vi "ge_XMLtoVarGrps.vi"(8 "error in":errorcluster, 10 "GXML String":string, 11 "ChanGroups":T1) -> (0 "error out":errorcluster, 2 "Speed Groups":T4[](array[typedef]))   [LabVIEW 2011]
uses:
  Custom Ctrls/Master Cfg/ge_ChanHeader.ctl
  Custom Ctrls/Master Cfg/ge_ChanDef.ctl
  Custom Ctrls/ge_MeasType.ctl
  Custom Ctrls/Master Cfg/ge_ChannelGroup.ctl
  Custom Ctrls/Master Cfg/ge_ChanVoltageCfg.ctl
  Custom Ctrls/Master CfgXML/ge_VoltChan.ctl
  Custom Ctrls/Master CfgXML/ge_VoltGroup.ctl
  Custom Ctrls/Master Cfg/ge_ChanDynamicCfg.ctl
  Custom Ctrls/Master CfgXML/ge_DyanChan.ctl
  Custom Ctrls/Master CfgXML/ge_DynGroup.ctl
  Custom Ctrls/Master Cfg/ge_ChanThrmcplCfg.ctl
  Custom Ctrls/Master CfgXML/ge_ThrmcplChan.ctl
  Custom Ctrls/Master CfgXML/ge_ThrmcplGroup.ctl
  Custom Ctrls/Master Cfg/ge_ChanRTDCfg.ctl
  Custom Ctrls/Master CfgXML/ge_RTDChan.ctl
  Custom Ctrls/Master CfgXML/ge_RTDGroup.ctl
  Custom Ctrls/Master Cfg/ge_ChanStrainCfg.ctl
  Custom Ctrls/Master CfgXML/ge_StrainChan.ctl
  Custom Ctrls/Master CfgXML/ge_StrainGroup.ctl
  Custom Ctrls/Master CfgXML/ge_CurrentChan.ctl
  Custom Ctrls/Master CfgXML/ge_CurrentGroup.ctl
  Custom Ctrls/Master Cfg/ge_ChanResCfg.ctl
  Custom Ctrls/Master CfgXML/ge_ResChan.ctl
  Custom Ctrls/Master CfgXML/ge_ResGroup.ctl
  Custom Ctrls/Master Cfg/ge_ChanFreqCfg.ctl
  Custom Ctrls/Master CfgXML/ge_FreqChan.ctl
  Custom Ctrls/Master CfgXML/ge_FreqGroup.ctl
  Custom Ctrls/Master Cfg/ge_ChanCurrentCfg.ctl
  Custom Ctrls/Master CfgXML/ge_TachGroup.ctl
  Custom Ctrls/Master CfgXML/ge_TachChan.ctl
  Custom Ctrls/Master Cfg/ge_ChanTachCfg.ctl
  Custom Ctrls/Master Cfg/ge_TachProcess.ctl
  Classes/Channel/Channel.lvclass
  Custom Ctrls/Master Cfg/ge_GrpHdr.ctl
  Custom Ctrls/Master CfgXML/ge_XMLHdr_ChanGroups.ctl
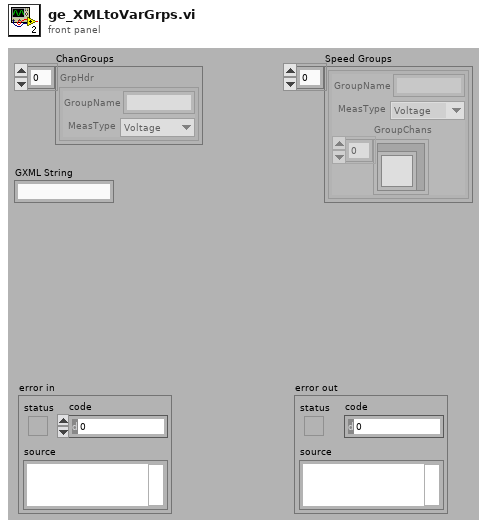
[diagram p1: front panel]
types:
  T1 = typedef "ge_XMLHdr_ChanGroups.ctl" = T2[]
  T2 = typedef "ge_GrpHdr.ctl" = cluster{"GroupName":string, "MeasType":T3}
  T3 = typedef "ge_MeasType.ctl" = enum16{"Voltage", "Frequency", "Tachometer", "Dynamic", "Thermocouple", "RTD", "Strain", "Current", "Resistance"}
  T4 = typedef "ge_ChannelGroup.ctl" = cluster{"GroupName":string, "MeasType":T3, "GroupChans":refnum<class "Channel.lvclass">[]}
  T5 = typedef "ge_VoltGroup.ctl" = cluster{"GroupName":string, "MeasType":T3, "GroupMems":T6[]}
  T6 = typedef "ge_VoltChan.ctl" = cluster{"ChanHdr":T7, "VoltChanCfg":T8}
  T7 = typedef "ge_ChanHeader.ctl" = cluster{"ChanName":string, "Alias":string, "ModbusAddr":string, "Device":string, "ToModBus":bool}
  T8 = typedef "ge_ChanVoltageCfg.ctl" = cluster{"VRange":dbl, "Term Cfg":u16, "Coupling":u16, "Scale":dbl, "Offset":dbl, "Unit_EU":string}
  T9 = typedef "ge_ChanDef.ctl" = cluster{"ChanHdr":T7, "ChanCfg":variant}
  T10 = typedef "ge_FreqGroup.ctl" = cluster{"GroupName":string, "MeasType":T3, "GroupMems":T11[]}
  T11 = typedef "ge_FreqChan.ctl" = cluster{"ChanHdr":T7, "FreqChanCfg":T12}
  T12 = typedef "ge_ChanFreqCfg.ctl" = cluster{"VRange":dbl, "Term Cfg":u16, "Coupling":u16, "Thresh":dbl, "Slope":u16, "Min EU":dbl, "Scale":dbl, "Offset":dbl, "Unit_EU":string}
  T13 = typedef "ge_TachGroup.ctl" = cluster{"GroupName":string, "MeasType":T3, "GroupMems":T14[]}
  T14 = typedef "ge_TachChan.ctl" = cluster{"ChanHdr":T7, "TachChanCfg":T15}
  T15 = typedef "ge_ChanTachCfg.ctl" = cluster{"VRange":dbl, "Term Cfg":u16, "Coupling":u16, "Unit_EU":string, "TachProc":T16}
  T16 = typedef "ge_TachProcess.ctl" = cluster{"PPR":dbl, "Thresh_V":dbl, "Slope":u16, "MinRPM":dbl}
  T17 = typedef "ge_DynGroup.ctl" = cluster{"GroupName":string, "MeasType":T3, "GroupMems":T18[]}
  T18 = typedef "ge_DyanChan.ctl" = cluster{"ChanHdr":T7, "DynChanCfg":T19}
  T19 = typedef "ge_ChanDynamicCfg.ctl" = cluster{"Sensitivity":dbl, "Unit_EU":string, "Iex":dbl, "VRange":dbl, "dB":bool, "dB Ref":dbl, "Cal Mag":dbl, "Cal Units":u16}
  T20 = typedef "ge_ThrmcplGroup.ctl" = cluster{"GroupName":string, "MeasType":T3, "GroupMems":T21[]}
  T21 = typedef "ge_ThrmcplChan.ctl" = cluster{"ChanHdr":T7, "ThrmcplChanCfg":T22}
  T22 = typedef "ge_ChanThrmcplCfg.ctl" = cluster{"Units":u16, "Type":u16, "cjc source":u16, "cjc val":dbl, "Scale":dbl, "Offset":dbl, "Approx Max":i32, "Approx Min":i32}
  T23 = typedef "ge_RTDGroup.ctl" = cluster{"GroupName":string, "MeasType":T3, "GroupMems":T24[]}
  T24 = typedef "ge_RTDChan.ctl" = cluster{"ChanHdr":T7, "RTDChanCfg":T25}
  T25 = typedef "ge_ChanRTDCfg.ctl" = cluster{"Ro":u16, "Units":u16, "Type":u16, "WireCfg":u16, "Scale":dbl, "Offset":dbl, "Approx Max":i32, "Approx Min":i32}
  T26 = typedef "ge_StrainGroup.ctl" = cluster{"GroupName":string, "MeasType":T3, "GroupMems":T27[]}
  T27 = typedef "ge_StrainChan.ctl" = cluster{"ChanHdr":T7, "StrainChanCfg":T28}
  T28 = typedef "ge_ChanStrainCfg.ctl" = cluster{"Strain Mode":u16, "Vex":dbl, "Bridge Type":u16, "GF":dbl, "Gauge Res":i32, "Poisson":dbl, "Lead Res":dbl, "Init uStrain":dbl, "GAF":dbl, "Approx Max":dbl, "Approx Min":dbl}
  T29 = typedef "ge_CurrentGroup.ctl" = cluster{"GroupName":string, "MeasType":T3, "GroupMems":T30[]}
  T30 = typedef "ge_CurrentChan.ctl" = cluster{"ChanHdr":T7, "CurrentChanCfg":T31}
  T31 = typedef "ge_ChanCurrentCfg.ctl" = cluster{"IRange":dbl, "Scale":dbl, "Offset":dbl, "Unit_EU":string}
  T32 = typedef "ge_ResGroup.ctl" = cluster{"GroupName":string, "MeasType":T3, "GroupMems":T33[]}
  T33 = typedef "ge_ResChan.ctl" = cluster{"ChanHdr":T7, "ResChanCfg":T34}
  T34 = typedef "ge_ChanResCfg.ctl" = cluster{"ORange":u16, "WireCfg":u16, "Scale":dbl, "Offset":dbl, "Unit_EU":string}
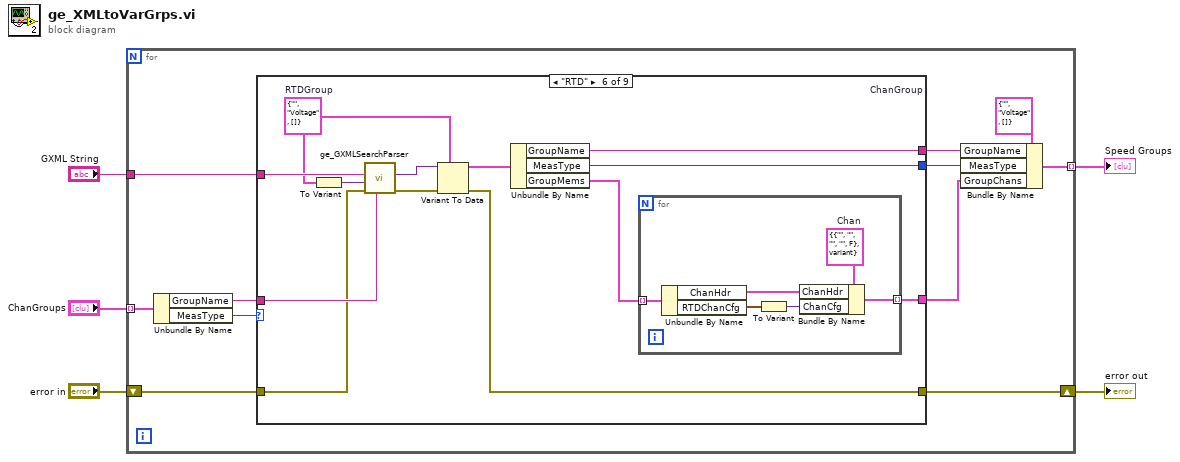
[diagram p0: block diagram]
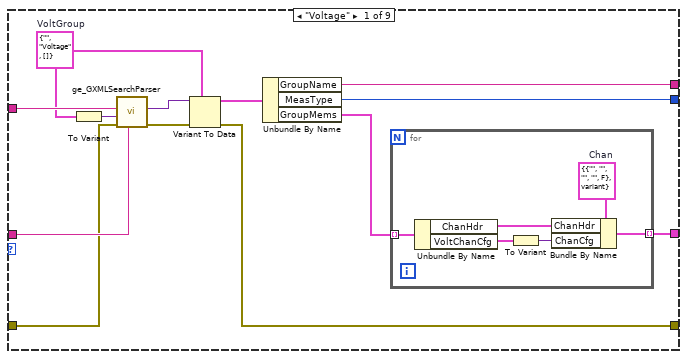
[diagram p2: hidden frame]
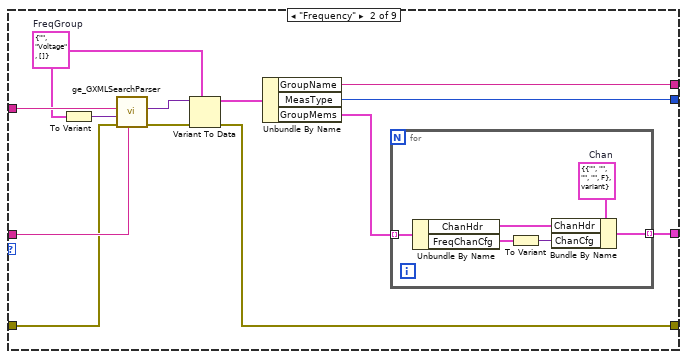
[diagram p3: hidden frame]
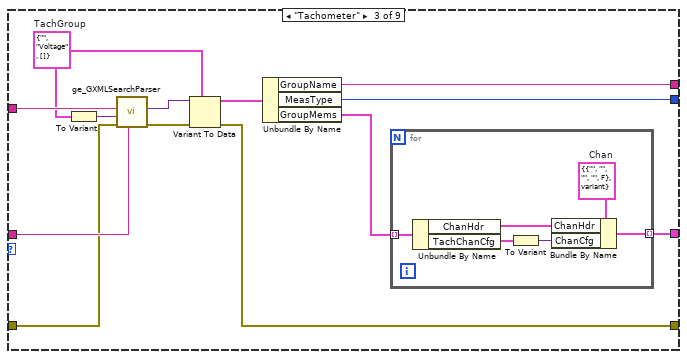
[diagram p4: hidden frame]
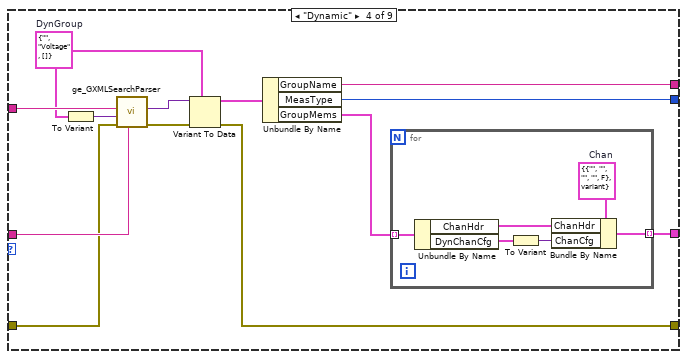
[diagram p5: hidden frame]
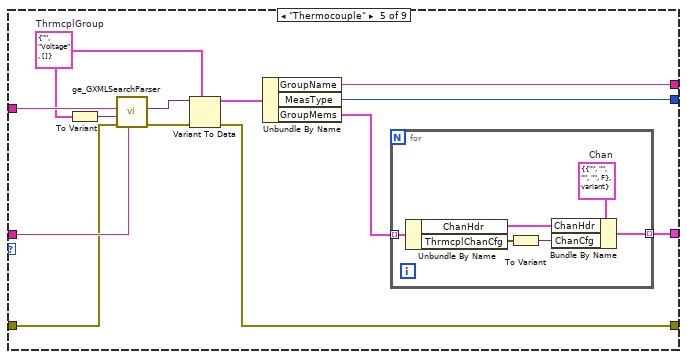
[diagram p6: hidden frame]
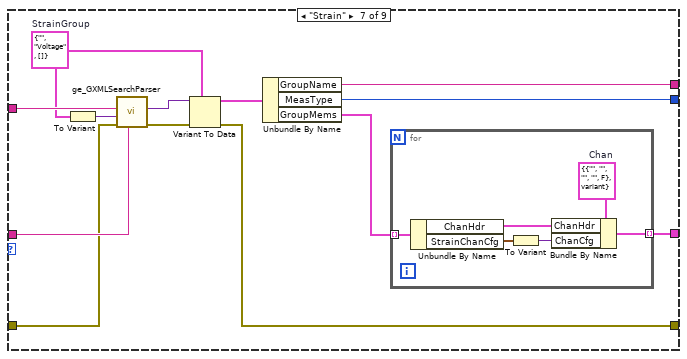
[diagram p7: hidden frame]
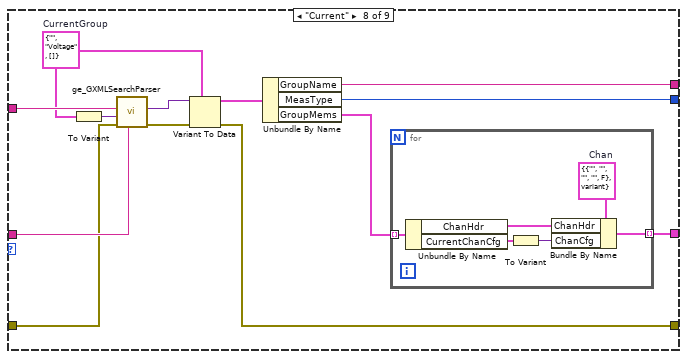
[diagram p8: hidden frame]
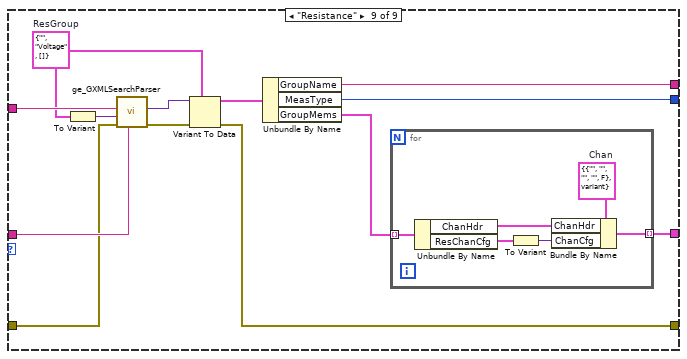
[diagram p9: hidden frame]
diagram:
  n1 = for {
    tunnel: "ChanGroups" -> [w16] mode=indexing
    tunnel: "GXML String" -> [w14]
    shift-right: [w12] -> w5
    shift-left: "error in" -> [w13]
    tunnel: [w6] -> w4 mode=indexing
    w10 = T4 {"GroupName"="", "MeasType"=enum."Voltage", "GroupChans"=[]}  # ChanGroup
    n2 = Unbundle By Name(w16) -> ("GroupName"=w15:string, "MeasType"=w11:T3)
    n3 = case shown="\"RTD\"" w11 {
      tunnel: w15 -> [w29 w48 w67 w86 w105 w124 w143 w162 w181]
      tunnel: w14 -> [w28 w47 w66 w85 w104 w123 w142 w161 w180]
      tunnel: w13 -> [w27 w46 w65 w84 w103 w122 w141 w160 w179]
      tunnel: [w24 w43 w62 w81 w100 w119 w138 w157 w176] -> w12
      tunnel: [w21 w40 w59 w78 w97 w116 w135 w154 w173] -> w9
      tunnel: [w20 w39 w58 w77 w96 w115 w134 w153 w172] -> w8
      tunnel: [w19 w38 w57 w76 w95 w114 w133 w152 w171] -> w7
      frame "Voltage" {
        w17 = T5 {"GroupName"="", "MeasType"=enum."Voltage", "GroupMems"=[]}  # VoltGroup
        n4 = To Variant(anything=w17) -> (Variant=w18:variant)
        n5 = call "ge_GXMLSearchParser.vi"("String ID"=w29, "error in"=w27, "TypeDesc"=w18, "XML String In"=w28) -> ("error out"=w25:errorcluster, "Parsed Data"=w26:variant)  [unwired: 6 in]
        n6 = Variant To Data(error in=w25, type=w17, Variant=w26) -> (data=w23:T5, error out=w24:errorcluster)
        n7 = Unbundle By Name(w23) -> ("GroupName"=w21:string, "MeasType"=w20:T3, "GroupMems"=w22:T6[])
        n8 = for {
          tunnel: w22 -> [w35] mode=indexing
          tunnel: [w30] -> w19 mode=indexing
          w33 = T9 {"ChanHdr"={"ChanName"="", "Alias"="", "ModbusAddr"="", "Device"="", "ToModBus"=FALSE}, "ChanCfg"=variant}  # Chan
          n9 = Unbundle By Name(w35) -> ("ChanHdr"=w32:T7, "VoltChanCfg"=w34:T8)
          n10 = To Variant(anything=w34) -> (Variant=w31:variant)
          n11 = Bundle By Name(cluster=w33, "ChanHdr"=w32, "ChanCfg"=w31) -> (w30:T9)
        }
      }
      frame "Frequency" {
        w36 = T10 {"GroupName"="", "MeasType"=enum."Voltage", "GroupMems"=[]}  # FreqGroup
        n12 = To Variant(anything=w36) -> (Variant=w37:variant)
        n13 = call "ge_GXMLSearchParser.vi"("String ID"=w48, "error in"=w46, "TypeDesc"=w37, "XML String In"=w47) -> ("error out"=w44:errorcluster, "Parsed Data"=w45:variant)  [unwired: 6 in]
        n14 = Variant To Data(error in=w44, type=w36, Variant=w45) -> (data=w42:T10, error out=w43:errorcluster)
        n15 = Unbundle By Name(w42) -> ("GroupName"=w40:string, "MeasType"=w39:T3, "GroupMems"=w41:T11[])
        n16 = for {
          tunnel: w41 -> [w54] mode=indexing
          tunnel: [w49] -> w38 mode=indexing
          w52 = T9 {"ChanHdr"={"ChanName"="", "Alias"="", "ModbusAddr"="", "Device"="", "ToModBus"=FALSE}, "ChanCfg"=variant}  # Chan
          n17 = Unbundle By Name(w54) -> ("ChanHdr"=w51:T7, "FreqChanCfg"=w53:T12)
          n18 = To Variant(anything=w53) -> (Variant=w50:variant)
          n19 = Bundle By Name(cluster=w52, "ChanHdr"=w51, "ChanCfg"=w50) -> (w49:T9)
        }
      }
      frame "Tachometer" {
        w55 = T13 {"GroupName"="", "MeasType"=enum."Voltage", "GroupMems"=[]}  # TachGroup
        n20 = To Variant(anything=w55) -> (Variant=w56:variant)
        n21 = call "ge_GXMLSearchParser.vi"("String ID"=w67, "error in"=w65, "TypeDesc"=w56, "XML String In"=w66) -> ("error out"=w63:errorcluster, "Parsed Data"=w64:variant)  [unwired: 6 in]
        n22 = Variant To Data(error in=w63, type=w55, Variant=w64) -> (data=w61:T13, error out=w62:errorcluster)
        n23 = Unbundle By Name(w61) -> ("GroupName"=w59:string, "MeasType"=w58:T3, "GroupMems"=w60:T14[])
        n24 = for {
          tunnel: w60 -> [w73] mode=indexing
          tunnel: [w68] -> w57 mode=indexing
          w71 = T9 {"ChanHdr"={"ChanName"="", "Alias"="", "ModbusAddr"="", "Device"="", "ToModBus"=FALSE}, "ChanCfg"=variant}  # Chan
          n25 = Unbundle By Name(w73) -> ("ChanHdr"=w70:T7, "TachChanCfg"=w72:T15)
          n26 = To Variant(anything=w72) -> (Variant=w69:variant)
          n27 = Bundle By Name(cluster=w71, "ChanHdr"=w70, "ChanCfg"=w69) -> (w68:T9)
        }
      }
      frame "Dynamic" {
        w74 = T17 {"GroupName"="", "MeasType"=enum."Voltage", "GroupMems"=[]}  # DynGroup
        n28 = To Variant(anything=w74) -> (Variant=w75:variant)
        n29 = call "ge_GXMLSearchParser.vi"("String ID"=w86, "error in"=w84, "TypeDesc"=w75, "XML String In"=w85) -> ("error out"=w82:errorcluster, "Parsed Data"=w83:variant)  [unwired: 6 in]
        n30 = Variant To Data(error in=w82, type=w74, Variant=w83) -> (data=w80:T17, error out=w81:errorcluster)
        n31 = Unbundle By Name(w80) -> ("GroupName"=w78:string, "MeasType"=w77:T3, "GroupMems"=w79:T18[])
        n32 = for {
          tunnel: w79 -> [w92] mode=indexing
          tunnel: [w87] -> w76 mode=indexing
          w90 = T9 {"ChanHdr"={"ChanName"="", "Alias"="", "ModbusAddr"="", "Device"="", "ToModBus"=FALSE}, "ChanCfg"=variant}  # Chan
          n33 = Unbundle By Name(w92) -> ("ChanHdr"=w89:T7, "DynChanCfg"=w91:T19)
          n34 = To Variant(anything=w91) -> (Variant=w88:variant)
          n35 = Bundle By Name(cluster=w90, "ChanHdr"=w89, "ChanCfg"=w88) -> (w87:T9)
        }
      }
      frame "Thermocouple" {
        w93 = T20 {"GroupName"="", "MeasType"=enum."Voltage", "GroupMems"=[]}  # ThrmcplGroup
        n36 = To Variant(anything=w93) -> (Variant=w94:variant)
        n37 = call "ge_GXMLSearchParser.vi"("String ID"=w105, "error in"=w103, "TypeDesc"=w94, "XML String In"=w104) -> ("error out"=w101:errorcluster, "Parsed Data"=w102:variant)  [unwired: 6 in]
        n38 = Variant To Data(error in=w101, type=w93, Variant=w102) -> (data=w99:T20, error out=w100:errorcluster)
        n39 = Unbundle By Name(w99) -> ("GroupName"=w97:string, "MeasType"=w96:T3, "GroupMems"=w98:T21[])
        n40 = for {
          tunnel: w98 -> [w111] mode=indexing
          tunnel: [w106] -> w95 mode=indexing
          w109 = T9 {"ChanHdr"={"ChanName"="", "Alias"="", "ModbusAddr"="", "Device"="", "ToModBus"=FALSE}, "ChanCfg"=variant}  # Chan
          n41 = Unbundle By Name(w111) -> ("ChanHdr"=w108:T7, "ThrmcplChanCfg"=w110:T22)
          n42 = To Variant(anything=w110) -> (Variant=w107:variant)
          n43 = Bundle By Name(cluster=w109, "ChanHdr"=w108, "ChanCfg"=w107) -> (w106:T9)
        }
      }
      frame "RTD" {
        w112 = T23 {"GroupName"="", "MeasType"=enum."Voltage", "GroupMems"=[]}  # RTDGroup
        n44 = To Variant(anything=w112) -> (Variant=w113:variant)
        n45 = call "ge_GXMLSearchParser.vi"("String ID"=w124, "error in"=w122, "TypeDesc"=w113, "XML String In"=w123) -> ("error out"=w120:errorcluster, "Parsed Data"=w121:variant)  [unwired: 6 in]
        n46 = Variant To Data(error in=w120, type=w112, Variant=w121) -> (data=w118:T23, error out=w119:errorcluster)
        n47 = Unbundle By Name(w118) -> ("GroupName"=w116:string, "MeasType"=w115:T3, "GroupMems"=w117:T24[])
        n48 = for {
          tunnel: w117 -> [w130] mode=indexing
          tunnel: [w125] -> w114 mode=indexing
          w128 = T9 {"ChanHdr"={"ChanName"="", "Alias"="", "ModbusAddr"="", "Device"="", "ToModBus"=FALSE}, "ChanCfg"=variant}  # Chan
          n49 = Unbundle By Name(w130) -> ("ChanHdr"=w127:T7, "RTDChanCfg"=w129:T25)
          n50 = To Variant(anything=w129) -> (Variant=w126:variant)
          n51 = Bundle By Name(cluster=w128, "ChanHdr"=w127, "ChanCfg"=w126) -> (w125:T9)
        }
      }
      frame "Strain" {
        w131 = T26 {"GroupName"="", "MeasType"=enum."Voltage", "GroupMems"=[]}  # StrainGroup
        n52 = To Variant(anything=w131) -> (Variant=w132:variant)
        n53 = call "ge_GXMLSearchParser.vi"("String ID"=w143, "error in"=w141, "TypeDesc"=w132, "XML String In"=w142) -> ("error out"=w139:errorcluster, "Parsed Data"=w140:variant)  [unwired: 6 in]
        n54 = Variant To Data(error in=w139, type=w131, Variant=w140) -> (data=w137:T26, error out=w138:errorcluster)
        n55 = Unbundle By Name(w137) -> ("GroupName"=w135:string, "MeasType"=w134:T3, "GroupMems"=w136:T27[])
        n56 = for {
          tunnel: w136 -> [w149] mode=indexing
          tunnel: [w144] -> w133 mode=indexing
          w147 = T9 {"ChanHdr"={"ChanName"="", "Alias"="", "ModbusAddr"="", "Device"="", "ToModBus"=FALSE}, "ChanCfg"=variant}  # Chan
          n57 = Unbundle By Name(w149) -> ("ChanHdr"=w146:T7, "StrainChanCfg"=w148:T28)
          n58 = To Variant(anything=w148) -> (Variant=w145:variant)
          n59 = Bundle By Name(cluster=w147, "ChanHdr"=w146, "ChanCfg"=w145) -> (w144:T9)
        }
      }
      frame "Current" {
        w150 = T29 {"GroupName"="", "MeasType"=enum."Voltage", "GroupMems"=[]}  # CurrentGroup
        n60 = To Variant(anything=w150) -> (Variant=w151:variant)
        n61 = call "ge_GXMLSearchParser.vi"("String ID"=w162, "error in"=w160, "TypeDesc"=w151, "XML String In"=w161) -> ("error out"=w158:errorcluster, "Parsed Data"=w159:variant)  [unwired: 6 in]
        n62 = Variant To Data(error in=w158, type=w150, Variant=w159) -> (data=w156:T29, error out=w157:errorcluster)
        n63 = Unbundle By Name(w156) -> ("GroupName"=w154:string, "MeasType"=w153:T3, "GroupMems"=w155:T30[])
        n64 = for {
          tunnel: w155 -> [w168] mode=indexing
          tunnel: [w163] -> w152 mode=indexing
          w166 = T9 {"ChanHdr"={"ChanName"="", "Alias"="", "ModbusAddr"="", "Device"="", "ToModBus"=FALSE}, "ChanCfg"=variant}  # Chan
          n65 = Unbundle By Name(w168) -> ("ChanHdr"=w165:T7, "CurrentChanCfg"=w167:T31)
          n66 = To Variant(anything=w167) -> (Variant=w164:variant)
          n67 = Bundle By Name(cluster=w166, "ChanHdr"=w165, "ChanCfg"=w164) -> (w163:T9)
        }
      }
      frame "Resistance" {
        w169 = T32 {"GroupName"="", "MeasType"=enum."Voltage", "GroupMems"=[]}  # ResGroup
        n68 = To Variant(anything=w169) -> (Variant=w170:variant)
        n69 = call "ge_GXMLSearchParser.vi"("String ID"=w181, "error in"=w179, "TypeDesc"=w170, "XML String In"=w180) -> ("error out"=w177:errorcluster, "Parsed Data"=w178:variant)  [unwired: 6 in]
        n70 = Variant To Data(error in=w177, type=w169, Variant=w178) -> (data=w175:T32, error out=w176:errorcluster)
        n71 = Unbundle By Name(w175) -> ("GroupName"=w173:string, "MeasType"=w172:T3, "GroupMems"=w174:T33[])
        n72 = for {
          tunnel: w174 -> [w187] mode=indexing
          tunnel: [w182] -> w171 mode=indexing
          w185 = T9 {"ChanHdr"={"ChanName"="", "Alias"="", "ModbusAddr"="", "Device"="", "ToModBus"=FALSE}, "ChanCfg"=variant}  # Chan
          n73 = Unbundle By Name(w187) -> ("ChanHdr"=w184:T7, "ResChanCfg"=w186:T34)
          n74 = To Variant(anything=w186) -> (Variant=w183:variant)
          n75 = Bundle By Name(cluster=w185, "ChanHdr"=w184, "ChanCfg"=w183) -> (w182:T9)
        }
      }
    }
    n76 = Bundle By Name(cluster=w10, "GroupName"=w9, "MeasType"=w8, "GroupChans"=w7) -> (w6:T4)
  }
  "error out" <- w5
  "Speed Groups" <- w4
